vi "Calculate ROI component's time.vi"(9 "AOD fill time (us)":dbl=24.4, 11 "Normalised ROI setup":T1 {"Apparent Frame Size" format="%#_6f"; "Original FOV (um)" format="%#_6f"; "Pixels per miniscan" format="%#_6f"; "Dwell Time per pixel" format="%#_6f"; "Resolution" format="%#_6f"; "ROI group ID" format="%#_6f"; "Laser Power (%)" format="%#_6f"; "Zoom" format="%#_6f"; "Frame Size" format="%#_6f"; "Number of lines" format="%#_6f"; "Composite ID" format="%#_6f"; "Angle (deg)" format="%#_6f"; "ROI Time (ns)" format="%#_6f"; "ROI ID" format="%#_6f"; "Pixels in ROI" format="%#_6f"; "ROI index" format="%#_6f"; "Z stop" format="%#_6f"; "Y stop" format="%#_6f"; "X stop" format="%#_6f"; "Z start" format="%#_6f"; "X start" format="%#_6f"; "Y start" format="%#_6f"}) -> (3 "ROI component's time (us)":dbl)   [LabVIEW 2020]
uses:
  User Interface/Visualisation/Functional Imaging Viewer/Typedefs/ROI parameters data type.ctl
  Typedefs/ROI ID Enum.ctl
  Global Variables/General Globals.vi
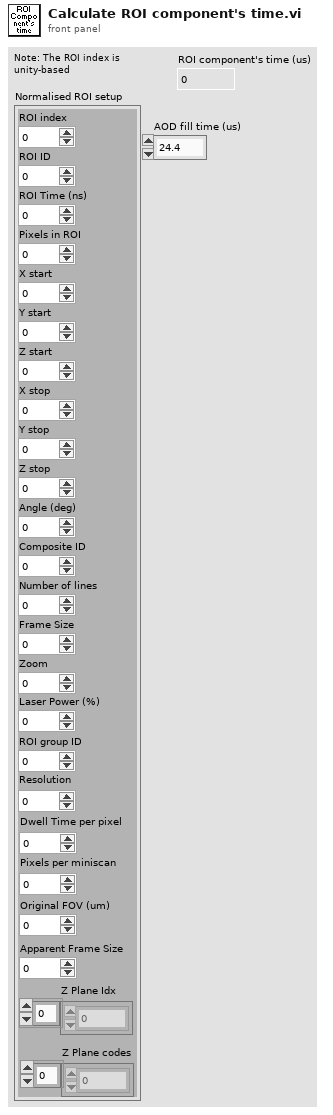
[diagram p1: front panel]
types:
  T1 = typedef "ROI parameters data type.ctl" = cluster{"ROI index":dbl, "ROI ID":dbl, "ROI Time (ns)":dbl, "Pixels in ROI":dbl, "X start":dbl, "Y start":dbl, "Z start":dbl, "X stop":dbl, "Y stop":dbl, "Z stop":dbl, "Angle (deg)":dbl, "Composite ID":dbl, "Number of lines":dbl, "Frame Size":dbl, "Zoom":dbl, "Laser Power (%)":dbl, "ROI group ID":dbl, "Resolution":dbl, "Dwell Time per pixel":dbl, "Pixels per miniscan":dbl, "Original FOV (um)":dbl, "Apparent Frame Size":dbl, "Z Plane Idx":i32[], "Z Plane codes":i32[]}
  T2 = typedef "ROI ID Enum.ctl" = enum16{"Point", "MiniScan", "Comp. MiniScan", "Rectangle", "Comp. volume", "Arb. plane point", "None"}
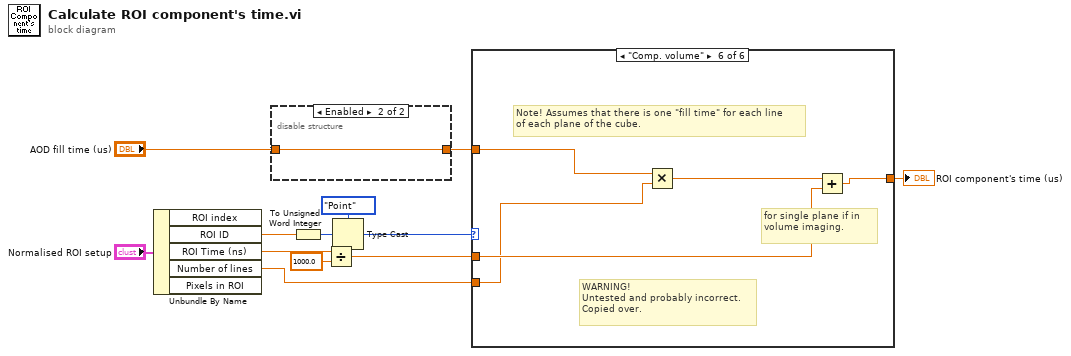
[diagram p0: block diagram]
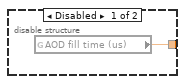
[diagram p2: hidden frame]
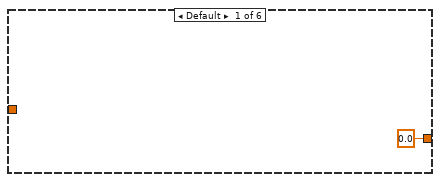
[diagram p3: hidden frame]
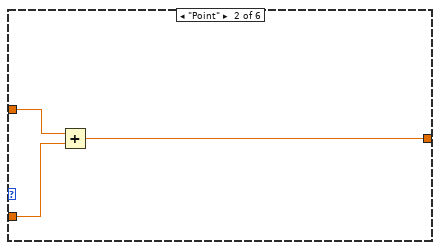
[diagram p4: hidden frame]
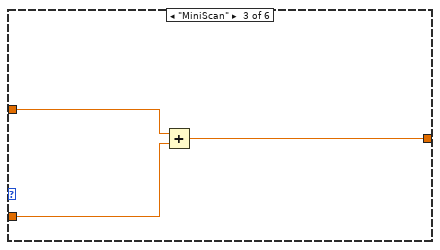
[diagram p5: hidden frame]
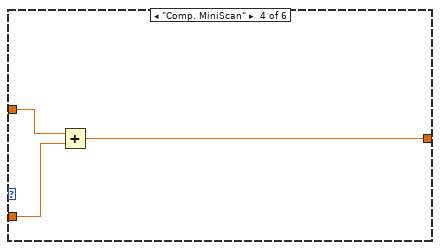
[diagram p6: hidden frame]
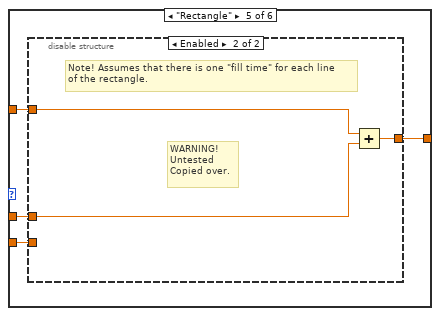
[diagram p7: hidden frame]
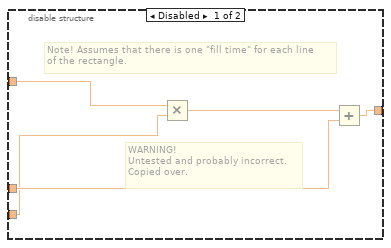
[diagram p8: hidden frame]
diagram:
  n1 = Unbundle By Name("Normalised ROI setup") -> ("ROI ID"=w2:dbl, "ROI Time (ns)"=w7:dbl, "Number of lines"=w9:dbl)  [unwired: 2 out]
  n2 = disable-structure shown="Enabled" {
    disable-tunnel: [w13 w14] -> w10
    disable-tunnel: "AOD fill time (us)" -> [_ w14]
    frame Disabled {
      n3 = global read "General Globals.vi" "AOD fill time (us)"() -> (w13:dbl)
    }
    frame Enabled {
    }
  }
  n4 = To Unsigned Word Integer(number=w2) -> (unsigned 16bit integer=w4:u16)
  n5 = Divide(x=w7, y=1000.0) -> (x/y=w8:dbl)
  n6 = Type Cast(type=ROI_ID_Enum."Point" ("ROI ID Enum"), x=w4) -> (*(type *) &x=w5:T2)
  n7 = case shown="\"Comp. volume\"" w5 {
    tunnel: w8 -> [_ w18 w21 w24 w28 w41]
    tunnel: w10 -> [_ w17 w20 w23 w27 w40]
    tunnel: [0.0 w16 w19 w22 w25 w37] -> w11
    tunnel: w9 -> [_ _ _ _ w26 w39]
    frame Default {
    }
    frame "Point" {
      n8 = Add(x=w17, y=w18) -> (x+y=w16:dbl)
    }
    frame "MiniScan" {
      n9 = Add(x=w20, y=w21) -> (x+y=w19:dbl)
    }
    frame "Comp. MiniScan" {
      n10 = Add(x=w23, y=w24) -> (x+y=w22:dbl)
    }
    frame "Rectangle" {
      n11 = disable-structure shown="Enabled" {
        disable-tunnel: w28 -> [w33 w36]
        disable-tunnel: w27 -> [w32 w34]
        disable-tunnel: w26 -> [w30 _]
        disable-tunnel: [w29 w35] -> w25
        frame Disabled {
          # "WARNING!\nUntested and probably incorrect.\nCopied over."
          # "Note! Assumes that there is one \"fill time\" for each line\nof the rectangle."
          n12 = Multiply(x=w32, y=w30) -> (x*y=w31:dbl)
          n13 = Add(x=w31, y=w33) -> (x+y=w29:dbl)
        }
        frame Enabled {
          # "WARNING!\nUntested\nCopied over."
          # "Note! Assumes that there is one \"fill time\" for each line\nof the rectangle."
          n14 = Add(x=w34, y=w36) -> (x+y=w35:dbl)
        }
      }
    }
    frame "Comp. volume" {
      # "WARNING!\nUntested and probably incorrect.\nCopied over."
      # "for single plane if in volume imaging."
      # "Note! Assumes that there is one \"fill time\" for each line\nof each plane of the cube."
      n15 = Multiply(x=w40, y=w39) -> (x*y=w38:dbl)
      n16 = Add(x=w38, y=w41) -> (x+y=w37:dbl)
    }
  }
  "ROI component's time (us)" <- w11
